vi "Replace Content.vi"(8 "error in (no error)":errorcluster, 10 "New Content":refnum<class "Debug Log.lvclass">, 11 "Debug Log in":refnum<class "Debug Log.lvclass">) -> (0 "error out":errorcluster, 3 "Debug Log out":refnum<class "Debug Log.lvclass">)   [LabVIEW 2020, in "Debug Log.lvclass"]
uses:
  Debug Log.lvclass
  Debug Log.lvclass/Debug Log.ctl
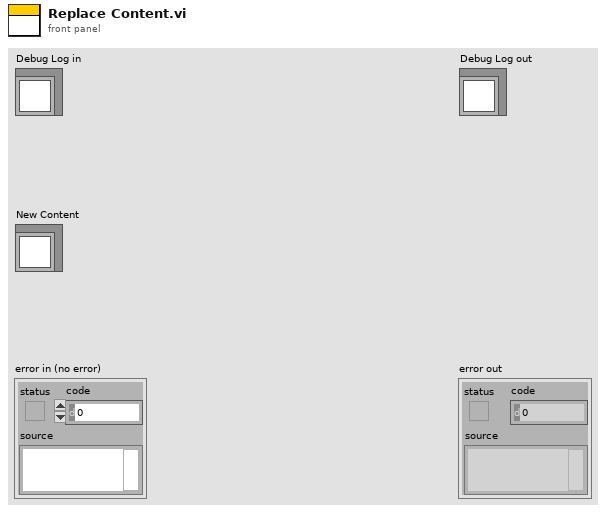
[diagram p1: front panel]
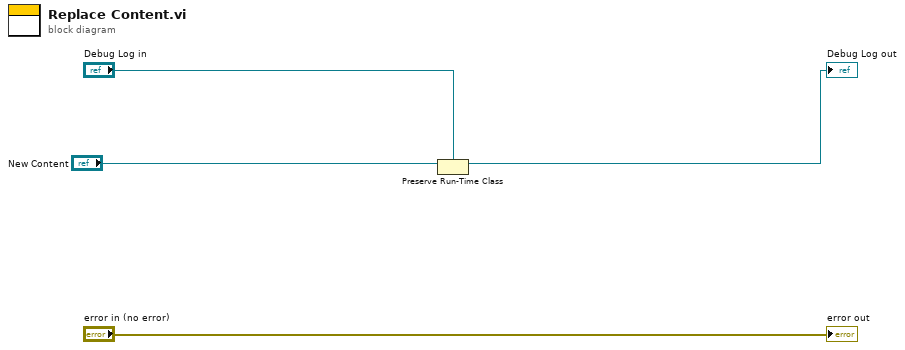
[diagram p0: block diagram]
diagram:
  n1 = Preserve Run-Time Class(object in="New Content", 2:"Debug Log in") -> (object out=→"Debug Log out":refnum<class "Debug Log.lvclass">)  [unwired: 1 in, 1 out]
  "error out" <- "error in (no error)"
